vi "PP.Encode.Decode.RC4.vi"(2 "Key (5 .. 256 Bytes)":string="123456", 3 "Text In":string="Hallo") -> (0 "Text Out":string)   [LabVIEW 2020, in "PixPack.lvlib"]
uses:
  PixPack.lvlib
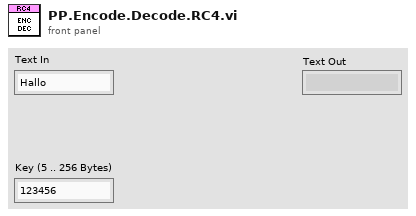
[diagram p1: front panel]
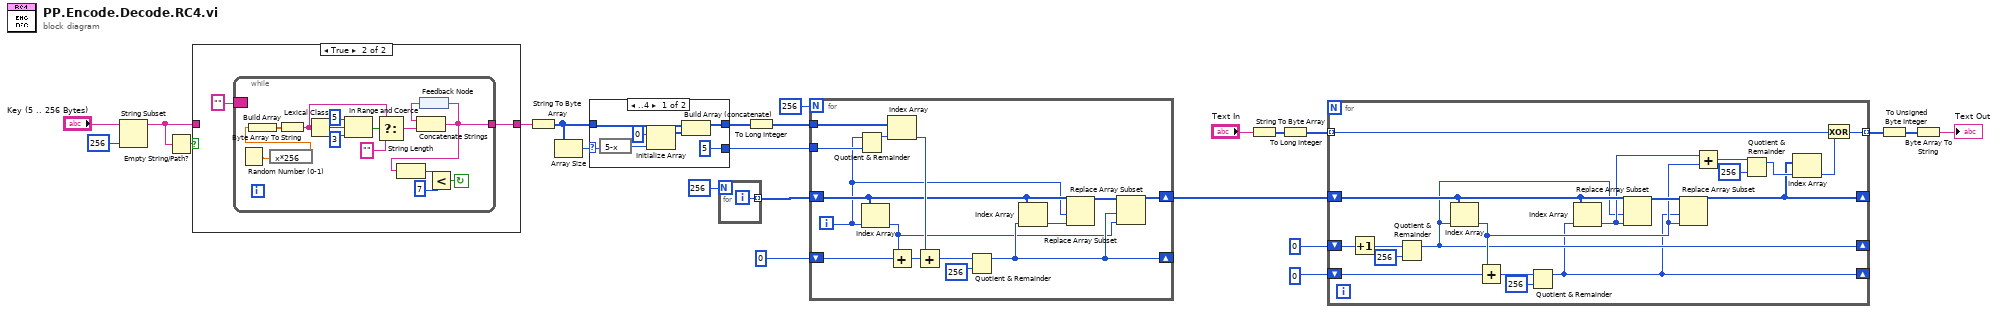
[diagram p0: block diagram]
diagram:
  n1 = String Subset(string="Key (5 .. 256 Bytes)", length (rest)=256 ("length (rest)")) -> (substring=w5:string)  [unwired: 1 in]
  n2 = Empty String/Path?(string/path=w5) -> (empty?=w6:bool)
  n3 = case shown="True" w6 {
    tunnel: [w24 w25] -> w4
    tunnel: w5 -> [w24 _]
    frame False {
    }
    frame True {
      n4 = while {
        tunnel: [w32] -> w25
        border: "" -> [_]
        stop <- w33 continue-if-true
        n5 = Random Number (0-1)() -> (number: 0 to 1=w41:dbl)
        n6 = expression code="x*256"(w41) -> (w40:dbl)
        n7 = Build Array(w40) -> (w39:dbl[])
        n8 = Byte Array To String(unsigned byte array=w39) -> (string=w31:string)
        n9 = Lexical Class(1:w31) -> (0:w30:i16)
        n10 = In Range and Coerce(upper limit=5, x=w30, lower limit=3) -> (In Range?=w27:bool)  [unwired: 1 out]
        n11 = Select(t=w31, s=w27, f="") -> (s? t:f=w37:string)
        n12 = feedback #1() -> (w36:string)
        n13 = Concatenate Strings(w36, w37) -> (w32:string)
        n14 = String Length(string=w32) -> (length=w35:i32)
        n15 = feedback-in #1(w32) -> ()
        n16 = Less?(x=w35, y=7) -> (x < y?=w33:bool)
      }
    }
  }
  n17 = String To Byte Array(string=w4) -> (unsigned byte array=w3:u8[])
  n18 = Array Size(array=w3) -> (size(s)=w19:i32)
  n19 = case shown="..4" w19 {
    selector: w19 -> [w48 w50]
    tunnel: [5 w50] -> w18
    tunnel: [w43 w49] -> w2
    tunnel: w3 -> [w44 w49]
    frame ..4 {
      n20 = expression code="5-x"(w48) -> (w46:i32)
      n21 = Initialize Array(u8 0 ("element"), w46) -> (w42:u8[])
      n22 = Build Array (concatenate)(w44, w42) -> (w43:u8[])
    }
    frame 5.. {
    }
  }
  n23 = for {
    N: 256 -> [_]
    tunnel: [w51] -> w20 mode=indexing
    i -> [w51]
  }
  n24 = To Long Integer(number=w2) -> (32bit integer=w1:i32[])
  n25 = for {
    N: 256 -> [_]
    shift-right: [w54] -> _
    shift-left: 0 -> [w66]
    tunnel: w18 -> [w65]
    tunnel: w1 -> [w62]
    shift-right: [w52] -> w11
    shift-left: w20 -> [w57]
    i -> [w56]
    n26 = Quotient & Remainder(x=w56, y=w65) -> (x-y*floor(x/y)=w61:i32)  [unwired: 1 out]
    n27 = Index Array(array=w57, index=w56) -> (element=w53:i32)
    n28 = Index Array(array=w62, index=w61) -> (element=w60:i32)
    n29 = Add(x=w53, y=w66) -> (x+y=w64:i32)
    n30 = Add(x=w60, y=w64) -> (x+y=w58:i32)
    n31 = Quotient & Remainder(x=w58, y=256) -> (x-y*floor(x/y)=w54:i32)  [unwired: 1 out]
    n32 = Index Array(array=w57, index=w54) -> (element=w55:i32)
    n33 = Replace Array Subset(array=w57, new element=w55, index=w56) -> (w63:i32[])
    n34 = Replace Array Subset(array=w63, new element=w53, index=w54) -> (w52:i32[])
  }
  n35 = String To Byte Array(string="Text In") -> (unsigned byte array=w16:u8[])
  n36 = To Long Integer(number=w16) -> (32bit integer=w13:i32[])
  n37 = for {
    shift-right: [w68] -> _
    shift-left: 0 -> [w85]
    shift-right: [w67] -> _
    shift-left: 0 -> [w82]
    shift-right: [w69] -> _
    shift-left: w11 -> [w79]
    tunnel: w13 -> [w72] mode=indexing
    tunnel: [w71] -> w12 mode=indexing
    n38 = Increment(x=w85) -> (x+1=w84:i32)
    n39 = Quotient & Remainder(x=w84, y=256) -> (x-y*floor(x/y)=w68:i32)  [unwired: 1 out]
    n40 = Index Array(array=w79, index=w68) -> (element=w77:i32)
    n41 = Add(x=w77, y=w82) -> (x+y=w80:i32)
    n42 = Quotient & Remainder(x=w80, y=256) -> (x-y*floor(x/y)=w67:i32)  [unwired: 1 out]
    n43 = Index Array(array=w79, index=w67) -> (element=w76:i32)
    n44 = Replace Array Subset(array=w79, new element=w76, index=w68) -> (w78:i32[])
    n45 = Replace Array Subset(array=w78, new element=w77, index=w67) -> (w69:i32[])
    n46 = Add(x=w76, y=w77) -> (x+y=w74:i32)
    n47 = Quotient & Remainder(x=w74, y=256) -> (x-y*floor(x/y)=w73:i32)  [unwired: 1 out]
    n48 = Index Array(array=w69, index=w73) -> (element=w70:i32)
    n49 = Exclusive Or(1:w70, 2:w72) -> (0:w71:i32)
  }
  n50 = To Unsigned Byte Integer(number=w12) -> (unsigned 8bit integer=w10:u8[])
  n51 = Byte Array To String(unsigned byte array=w10) -> (string=→"Text Out":string)
